vi "Test PWM Timing.vi"(8 "error in (no error)":errorcluster, 11 "TimedPWMControl in":refnum<class "TimedPWMControl.lvclass">) -> (0 "error out":errorcluster, 3 "TimedPWMControl out":refnum<class "TimedPWMControl.lvclass">)   [LabVIEW 2020, in "VolatusControl.lvlib" / "TimedPWMControl.lvclass"]
uses:
  TimedPWMControl.lvclass
  TimedPWMControl.lvclass/TimedPWMControl.ctl
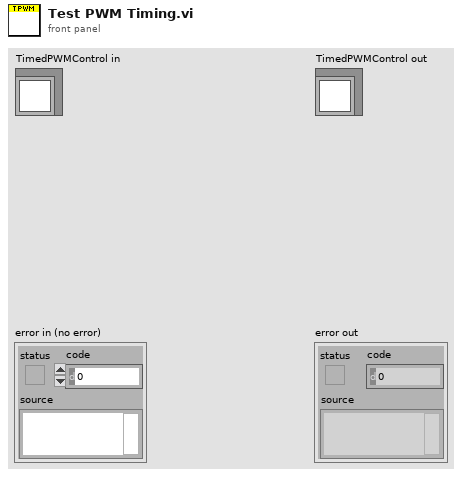
[diagram p1: front panel]
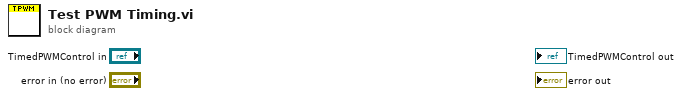
[diagram p0: block diagram]
diagram:
